vi "LOG Basic Data Log.vi"(0 "Directory Log Path":path, 2 "Header Text":string, 7 "Line To Append":string, 11 "Error in (no error)":errorcluster, 12 "Append Mode (new line)":T1=enum."New Line", 13 "Size Limit (250 KB)":dbl=250.0 format="%.2f", 14 "Timestamp (t:yes)":bool=TRUE) -> (4 "Logged Line":string, 6 "Current Files Size":dbl=250.0 format="%.2f", 8 "Current Logfile Path":path, 15 "Error out":errorcluster)   [LabVIEW 2011]
doc: "This VI is used for the purpose of logging data to a file. The \"Directory Log Name\" should contain the directory name that you want your log files to be placed. This directory MUST have a \"_\" (i.e., \"underscore\") contained in it. An example would be: BEESON_DIR. The VI checks to see if your directory is valid and then will name all of your logfiles \"BEESON_[n].log\" were \"n\" is a U32 integer pertaining to the order in which the file was created. A new logfile will dynamically be created based on the current logfile's size in comparison to the \"Size Limit.\" The most recent logfile will always be filled to capacity before the next one is created.\n\nIf files are deleted from the logfile directory in use then the vi will create a file next in the sequence of previously used numbers.\n\nThis scheme of logging data will support 4,294,967,295 files per directory, and at 250k a piece will top out at around 1,000 Tera-Bytes Maximum--well beyond any PCs capabilities! So delete old files before your disk becomes full.\n\nThis vi was created by David Gianetto, contact me with any problems, questions, etc."
uses:
  File IO/Type Defs/FILE New Line Enum.ctl
  File IO/Type Defs/FILE Append Mode Enum.ctl
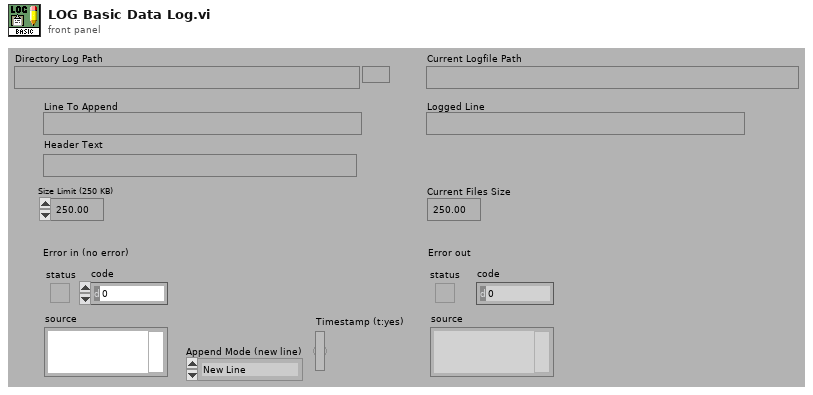
[diagram p1: front panel]
types:
  T1 = typedef "FILE New Line Enum.ctl" = enum16{"No New Line", "New Line"}
  T2 = typedef "FILE Append Mode Enum.ctl" = enum16{"Overwrite", "Append"}
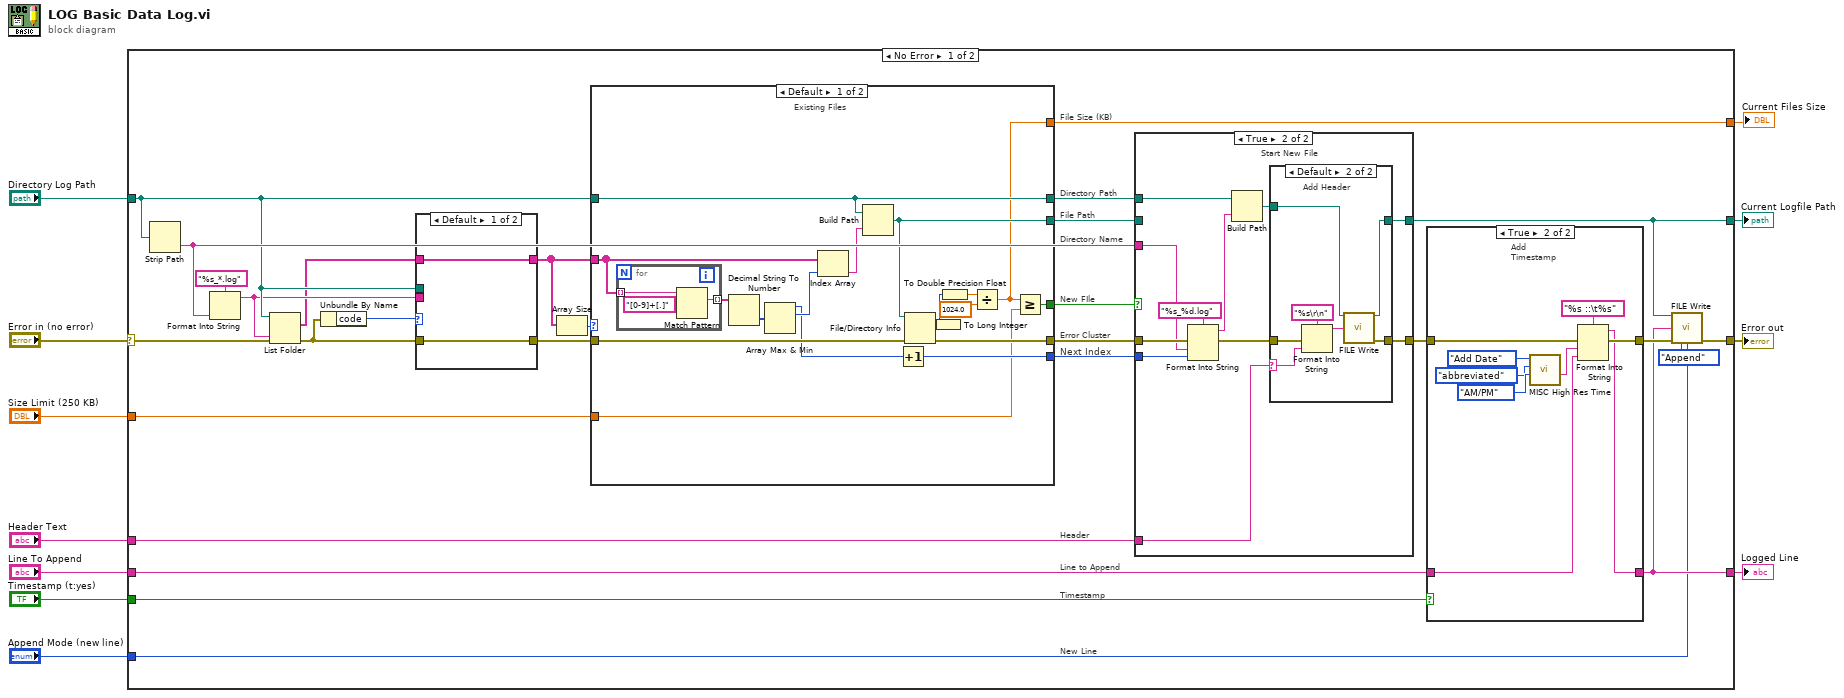
[diagram p0: block diagram]
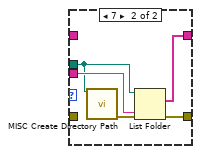
[diagram p2: hidden frame]
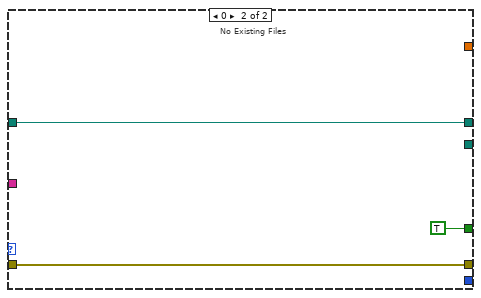
[diagram p4: hidden frame]
diagram:
  n1 = case shown="No Error" "Error in (no error)" {
    selector: "Error in (no error)" -> [w19 w104]
    tunnel: "Line To Append" -> [w36 _]
    tunnel: "Directory Log Path" -> [w15 w105]
    tunnel: "Size Limit (250 KB)" -> [w21 _]
    tunnel: [w31 w104] -> w10
    tunnel: [w35 _] -> w9
    tunnel: [w26 w105] -> w8
    tunnel: "Header Text" -> [w25 _]
    tunnel: [w30 _] -> w6
    tunnel: "Timestamp (t:yes)" -> [w24 _]
    tunnel: "Append Mode (new line)" -> [w29 _]
    frame No Error {
      # "New Line"
      # "Timestamp"
      # "Line to Append"
      # "Header"
      # "Next Index"
      # "Error Cluster"
      # "New FIle"
      # "Directory Name"
      # "File Path"
      # "Directory Path"
      # "File Size (KB)"
      n2 = Strip Path(path=w15) -> (name=w23:string)  [unwired: 1 out]
      n3 = Format Into String(format string="%s_*.log", w23) -> (resulting string=w14:string)  [unwired: 2 in, 1 out]
      n4 = List Folder(path=w15, pattern=w14, error in=w19) -> (filenames=w13:string[], error out=w16:errorcluster)  [unwired: 3 out]
      n5 = Unbundle By Name(w16) -> ("code"=w17:i32)
      n6 = case shown="Default" w17 {
        tunnel: [w41 w45] -> w18
        tunnel: w16 -> [w41 _]
        tunnel: w15 -> [_ w42]
        tunnel: w14 -> [_ w44]
        tunnel: [w40 w43] -> w12
        tunnel: w13 -> [w40 _]
        frame Default {
        }
        frame 7 {
          n7 = call "MISC Create Directory Path.vi"("Path"=w42) -> ("Error Out"=w46:errorcluster)  [unwired: 2 in, 12 out]
          n8 = List Folder(path=w42, pattern=w44, error in=w46) -> (filenames=w43:string[], error out=w45:errorcluster)  [unwired: 3 out]
        }
      }
      n9 = Array Size(array=w12) -> (size(s)=w27:i32)
      n10 = case shown="Default" w27 {
        tunnel: w12 -> [w68 _]
        tunnel: [w61 _] -> w35
        tunnel: [w75 w81] -> w34
        tunnel: w15 -> [w62 w80]
        tunnel: [w63 _] -> w37
        tunnel: [w67 _] -> w38
        tunnel: w18 -> [w74 w81]
        tunnel: [w62 w80] -> w22
        tunnel: w21 -> [w60 _]
        tunnel: [w59 TRUE] -> w20
        frame Default {
          # "Existing Files"
          n11 = for {
            tunnel: w68 -> [w78] mode=indexing
            tunnel: [w76] -> w66 mode=indexing
            n12 = Match Pattern(string=w78, regular expression="[0-9]+[.]") -> (match substring=w76:string)  [unwired: 4 out]
          }
          n13 = Decimal String To Number(string=w66) -> (number=w65:i32[])  [unwired: 3 out]
          n14 = Array Max & Min(array=w65) -> (max value=w64:i32, max index (indices)=w72:i32)  [unwired: 2 out]
          n15 = Index Array(array=w68, index=w72) -> (element=w73:string)
          n16 = Build Path(base path=w62, name or relative path=w73) -> (appended path=w67:path)
          n17 = Increment(x=w64) -> (x+1=w63:i32)
          n18 = File/Directory Info(path=w67, error in=w74) -> (size=w58:i64, error out=w75:errorcluster)  [unwired: 5 out]
          n19 = To Long Integer(number=w58) -> (32bit integer=w71:i32)
          n20 = To Double Precision Float(number=w71) -> (double precision float=w70:dbl)
          n21 = Divide(x=w70, y=1024.0) -> (x/y=w61:dbl)
          n22 = Greater Or Equal?(x=w61, y=w60) -> (x >= y?=w59:bool)
        }
        frame 0 {
          # "No Existing Files"
        }
      }
      n23 = case shown="True" w20 {
        tunnel: w38 -> [w83 _]
        tunnel: [w83 w92] -> w26
        tunnel: w37 -> [_ w87]
        tunnel: w23 -> [_ w89]
        tunnel: w25 -> [_ w88]
        tunnel: w34 -> [w82 w90]
        tunnel: [w82 w93] -> w33
        tunnel: w22 -> [_ w84]
        frame False {
          # "Append to Existing File"
        }
        frame True {
          # "Start New File"
          n24 = Format Into String(format string="%s_%d.log", error in=w90, w89, w87) -> (resulting string=w85:string, error out=w91:errorcluster)  [unwired: 1 in]
          n25 = Build Path(base path=w84, name or relative path=w85) -> (appended path=w94:path)
          n26 = case shown="Default" w88 {
            selector: w88 -> [_ w99]
            tunnel: w94 -> [w96 w103]
            tunnel: [w95 w102] -> w93
            tunnel: [w96 w101] -> w92
            tunnel: w91 -> [w95 w100]
            frame "" {
              # "No Header"
            }
            frame Default {
              # "Add Header"
              n27 = Format Into String(format string="%s\r\n", error in=w100, w99) -> (resulting string=w98:string)  [unwired: 1 in, 1 out]
              n28 = call "FILE Write.vi"("File Path (dialog if empty)"=w103, "Write String"=w98) -> ("New File Path"=w101:path, "Error Out"=w102:errorcluster)  [unwired: 9 in, 3 out]
            }
          }
        }
      }
      n29 = case shown="True" w24 {
        tunnel: w36 -> [w48 w57]
        tunnel: w33 -> [w47 w56]
        tunnel: [w47 w55] -> w32
        tunnel: [w48 w54] -> w30
        frame False {
          # "No\nTimestamp"
        }
        frame True {
          # "Add\nTimestamp"
          n30 = call "MISC High Res Time.vi"("Time Standard (am/pm)"=enum16{"AM/PM", "24 Hour"}."AM/PM", "Date Format (Abb)"=enum16{"short", "long", "abbreviated"}."abbreviated" ("date format (abbreviated)"), "Mode (add date)"=enum16{"Add Date", "Time Only"}."Add Date") -> ("Date/Time String"=w49:string)  [unwired: 6 out]
          n31 = Format Into String(format string="%s ::\t%s", error in=w56, w49, w57) -> (resulting string=w54:string, error out=w55:errorcluster)  [unwired: 1 in]
        }
      }
      n32 = call "FILE Write.vi"("File Path (dialog if empty)"=w26, "Write String"=w30, "Error In (no error)"=w32, "Append/Overwrite (Overwrite)"=FILE_Append_Mode_Enum."Append", "New Line on Append?"=w29) -> ("Error Out"=w31:errorcluster)  [unwired: 6 in, 4 out]
    }
    frame Error {
    }
  }
  "Error out" <- w10
  "Current Files Size" <- w9
  "Current Logfile Path" <- w8
  "Logged Line" <- w6
